vi "CAN USB Write flex prot leng.vi"(3 "CAN_Message":T1={"ID"=0, "MSG type"=enum."STD, NO RTR", "LEN"=0, "Data"=[0, 0, 0, 0, 0, 0, 0, 0]} {"ID" format="%.0x"}) -> (1 "Error Number":u32 format="%.0x")   [LabVIEW 2009]
doc: "CAN Write schreibt eine Nachricht in die Sende-Queue des Treibers. Rückgabe ist ein Fehlercode wie er in den Header-Dateien beschrieben ist."
uses:
  Pcan_usb.dll
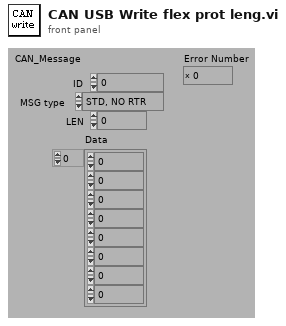
[diagram p1: front panel]
types:
  T1 = cluster{"ID":u32, "MSG type":enum8{"STD, NO RTR", "STD,RTR", "XTD, NO RTR", "XTD, RTR"}, "LEN":u8, "Data":u8[]}
  T2 = enum8{"STD, NO RTR", "STD,RTR", "XTD, NO RTR", "XTD, RTR"}
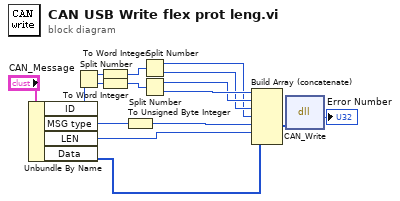
[diagram p0: block diagram]
diagram:
  n1 = Unbundle By Name("CAN_Message") -> ("ID"=w7:u32, "MSG type"=w4:T2, "LEN"=w5:u8, "Data"=w1:u8[])
  n2 = Split Number(x=w7) -> (hi(x)=w8:u16, lo(x)=w9:u16)
  n3 = To Word Integer(number=w8) -> (16bit integer=w11:i16)
  n4 = To Word Integer(number=w9) -> (16bit integer=w12:i16)
  n5 = To Unsigned Byte Integer(number=w4) -> (unsigned 8bit integer=w10:u8)
  n6 = Split Number(x=w11) -> (hi(x)=w13:u8, lo(x)=w14:u8)
  n7 = Split Number(x=w12) -> (hi(x)=w15:u8, lo(x)=w16:u8)
  n8 = Build Array (concatenate)(w16, w15, w14, w13, w10, w5, w1) -> (w3:u8[])
  n9 = dll-call lib="C:/Documents and Settings/PQ/Desktop/LabView-Dateien/PCAN_USB.dll" fn="CAN_Write"("TPCANMsg"=w3) -> ("Error Number"=→"Error Number":u32)  [unwired: 4 in, 2 out]
